vi "Electronics ON.vi"(1 "Electronics":bool) -> ()   [LabVIEW 2018]
uses:
  Type Defs/State Machine.ctl
  <vilib>/rvi/Emulation/niFpgaGetClockAttributes.vi
  <vilib>/rvi/Emulation/niFpgaSctlEmulationGetInTimedLoop.vi
  <vilib>/rvi/Emulation/niFpgaEmulationReportErrorSimple.vi
  <vilib>/rvi/eio/common/nirviEmuTemplateMethod_errors.vi
  <vilib>/rvi/Emulation/niFpgaCriticalErrorInLSC.vi
  <vilib>/eio/EIONode/EIONode.xnode
panel:
  # "Electronics ON/OFF"
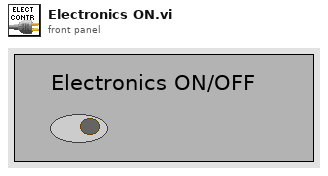
[diagram p1: front panel]
types:
  T1 = typedef "State Machine.ctl" = enum16{"Case 0", "Case 1", "Case 2", "Case 3", "Case 4", "Case 5", "Case 6", "Case 7", "Case 8", "Case 9", "Case 10", "Case 11", "Case 12", "Case 13", "Case 14", "Case 15", "Case 16", "Error", "Exit"}
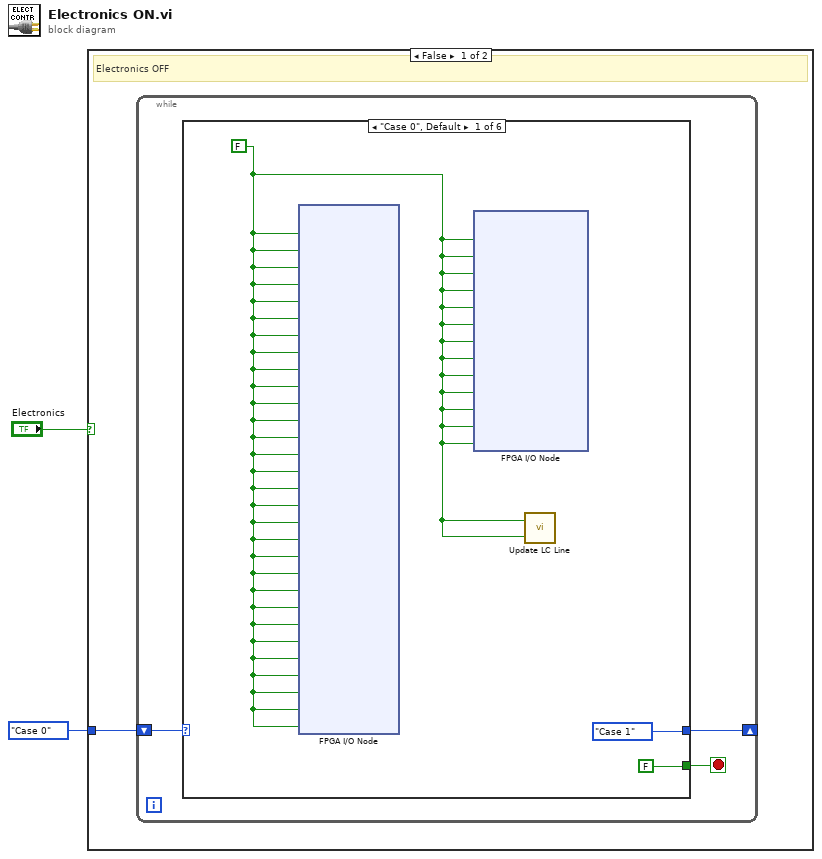
[diagram p0: block diagram]
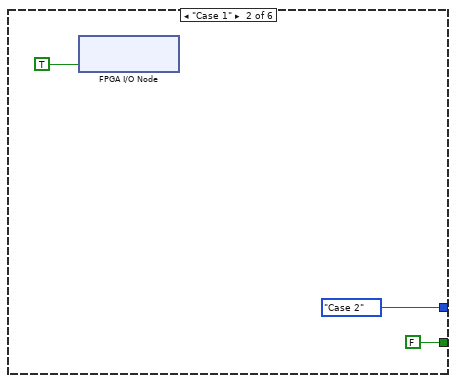
[diagram p2: hidden frame]
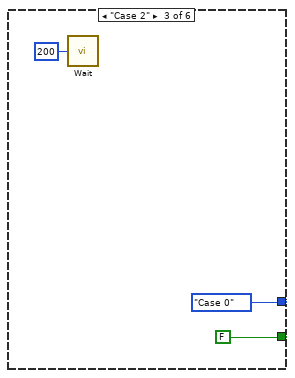
[diagram p3: hidden frame]
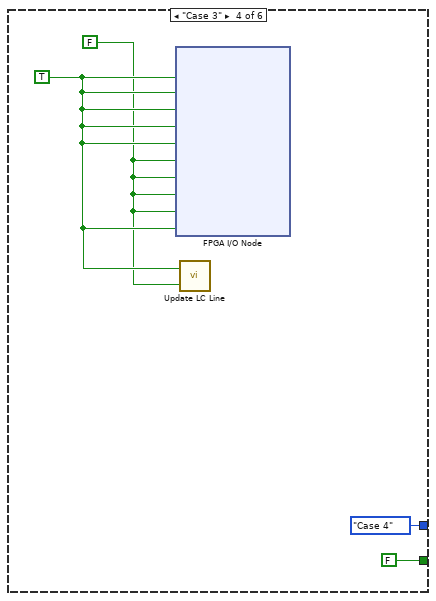
[diagram p4: hidden frame]
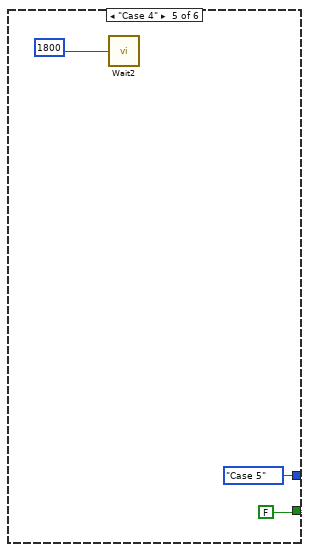
[diagram p5: hidden frame]
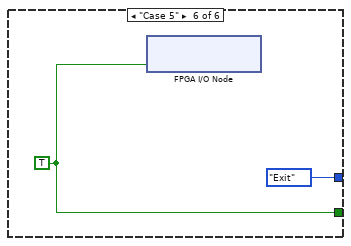
[diagram p6: hidden frame]
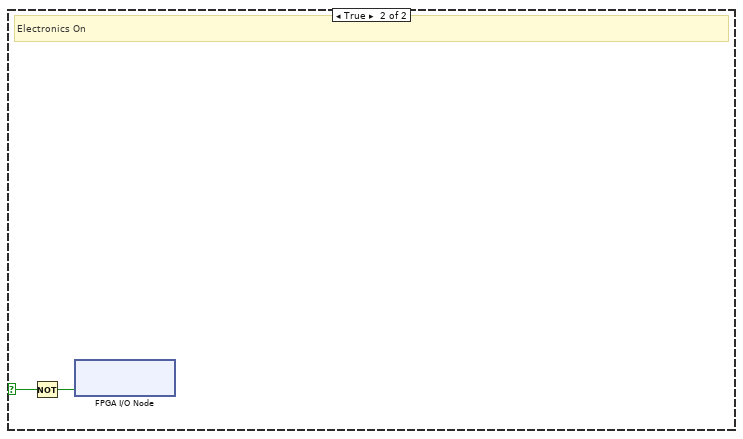
[diagram p7: hidden frame]
diagram:
  n1 = case shown="False" "Electronics" {
    selector: "Electronics" -> [_ w26]
    tunnel: State_Machine."Case 0" ("Enum") -> [w3 _]
    frame False {
      # "Electronics OFF"
      n2 = while {
        shift-right: [w4] -> _
        shift-left: w3 -> [w6]
        stop <- w5 stop-if-true
        n3 = case shown="\"Case 0\", Default" w6 {
          tunnel: [FALSE FALSE FALSE FALSE FALSE w23] -> w5
          tunnel: [State_Machine."Case 1" ("Enum") State_Machine."Case 2" ("Enum") State_Machine."Case 0" ("Enum") State_Machine."Case 4" ("Enum") State_Machine."Case 5" ("Enum") State_Machine."Exit" ("Enum")] -> w4
          frame "Case 0", Default {
            w7 = FALSE
            n4 = xnode "FPGA I/O Node"("MISO"=w7, "MOSI"=w7, "SCLK"=w7, "BS4"=w7, "BS3"=w7, "BS2"=w7, "BS1"=w7, "BS0"=w7, "CS2"=w7, "CS1"=w7, "CS0"=w7, "Electronics"=w7, "D17"=w7, "D16"=w7, "D15"=w7, "D14"=w7, "D13"=w7, "D12"=w7, "D11"=w7, "D10"=w7, "D9"=w7, "D8"=w7, "D7"=w7, "D6"=w7, "D5"=w7, "D4"=w7, "D3"=w7, "D2"=w7, "D1"=w7, "D0"=w7) -> ()  [unwired: 30 in, 30 out]
            n5 = xnode "FPGA I/O Node"("LDAC"=w7, "VAC CLK"=w7, "VAC CONVST"=w7, "LREG"=w7, "FSYNCH"=w7, "SpareOut"=w7, "DAC A1"=w7, "DAC A0"=w7, "DAC WR"=w7, "Filament B"=w7, "Filament C"=w7, "Filament E"=w7, "Reset"=w7) -> ()  [unwired: 13 in, 13 out]
            n6 = call "Update LC Line.vi"("LC Stop"=w7, "LC Hold"=w7) -> ()  [unwired: 1 in]
          }
          frame "Case 1" {
            n7 = xnode "FPGA I/O Node"("Electronics"=TRUE) -> ()  [unwired: 1 in, 1 out]
          }
          frame "Case 2" {
            n8 = call "Wait"("Count(mSec)"=u8 200) -> ()  [unwired: 1 out]
          }
          frame "Case 3" {
            w18 = TRUE
            w17 = FALSE
            n9 = xnode "FPGA I/O Node"("DAC A1"=w18, "DAC A0"=w18, "DAC WR"=w18, "Reset"=w18, "LDAC"=w18, "VAC CONVST"=w17, "VAC CLK"=w17, "Filament B"=w17, "Filament C"=w17, "Filament E"=w18) -> ()  [unwired: 10 in, 10 out]
            n10 = call "Update LC Line.vi"("LC Stop"=w17, "LC Hold"=w18) -> ()  [unwired: 1 in]
          }
          frame "Case 4" {
            n11 = call "Wait2"("Count(mSec)"=u16 1800) -> ()  [unwired: 1 out]
          }
          frame "Case 5" {
            w23 = TRUE ("RMC/DIO57")
            n12 = xnode "FPGA I/O Node"("VAC CONVST"=w23) -> ()  [unwired: 1 in, 1 out]
          }
        }
      }
    }
    frame True {
      # "Electronics On"
      n13 = Not(x=w26) -> (.not. x?=w25:bool)
      n14 = xnode "FPGA I/O Node"("Electronics"=w25) -> ()  [unwired: 1 in, 1 out]
    }
  }
